vi "SVT Pumps Fans.vi"(0 "nominal speed [RPM]":dbl=1200.0, 1 "desired units":u16(ring) items=["Hz", "Order"], 5 "number of blades":u32=3, 7 "number of diffuser vanes":u32=10, 9 "blade length":dbl=1.0, 11 "error in (no error)":errorcluster) -> (3 "blade tip speed":dbl=62.83185307179586, 4 "blade pass frequency":dbl=60.0, 6 "blade rate frequency":dbl=600.0, 14 "common factor":i32=1, 15 "error out":errorcluster)   [LabVIEW 2017, in "SoundVib_MachineCharacteristic.lvlib"]
doc: "Calculates characteristic frequencies or orders of flow-induced machinery, such as pumps and fans."
uses:
  <vilib>/addons/Sound and Vibration/svt_Machine Characteristic/SoundVib_MachineCharacteristic.lvlib
  <vilib>/gmath/NI_Gmath.lvlib
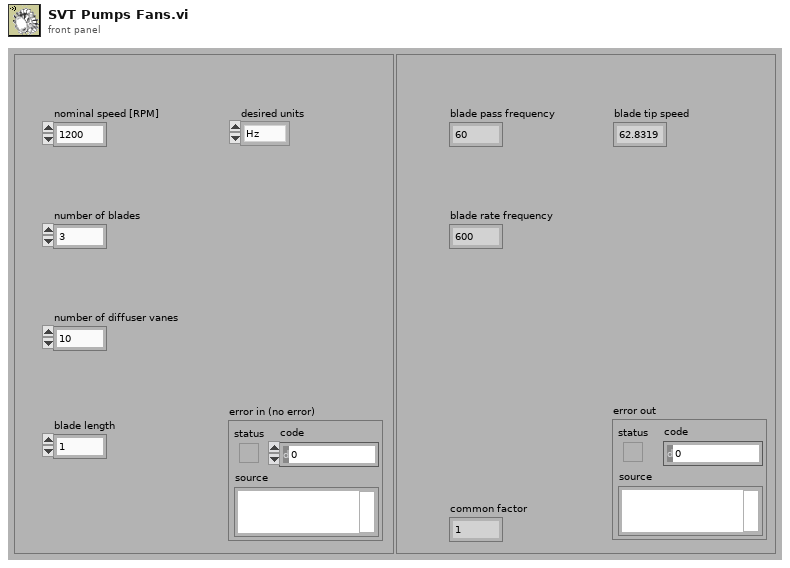
[diagram p1: front panel]
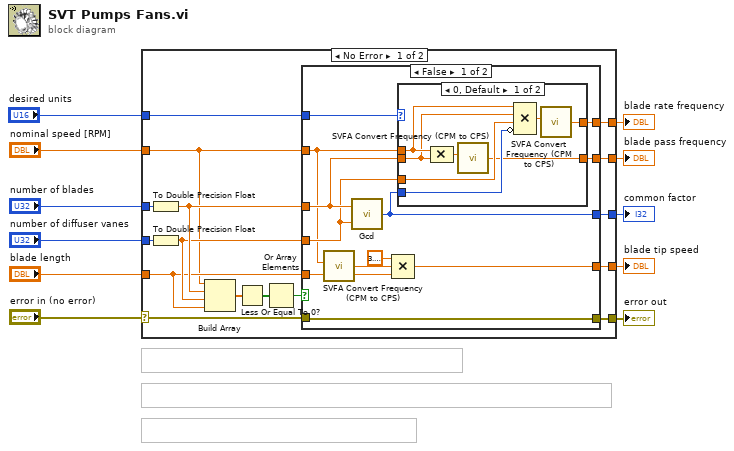
[diagram p0: block diagram]
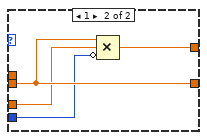
[diagram p2: hidden frame]
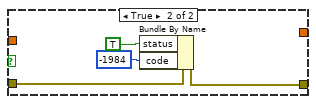
[diagram p3: hidden frame]
diagram:
  n1 = case shown="No Error" "error in (no error)" {
    selector: "error in (no error)" -> [w22 w56]
    tunnel: "blade length" -> [w18 _]
    tunnel: "number of diffuser vanes" -> [w27 _]
    tunnel: "number of blades" -> [w26 _]
    tunnel: "nominal speed [RPM]" -> [w15 _]
    tunnel: [w21 w56] -> w6
    tunnel: [w17 _] -> w5
    tunnel: "desired units" -> [w16 _]
    tunnel: [w14 _] -> w3
    tunnel: [w13 _] -> w2
    tunnel: [w12 _] -> w1
    frame No Error {
      n2 = To Double Precision Float(number=w26) -> (double precision float=w20:dbl)
      n3 = To Double Precision Float(number=w27) -> (double precision float=w19:dbl)
      n4 = Build Array(w15, w20, w19, w18) -> (w25:dbl[])
      n5 = Less Or Equal To 0?(x=w25) -> (x <= 0?=w24:bool[])
      n6 = Or Array Elements(Boolean array=w24) -> (logical OR=w23:bool)
      n7 = case shown="False" w23 {
        tunnel: w22 -> [w31 w55]
        tunnel: [w31 w54] -> w21
        tunnel: w20 -> [w38 _]
        tunnel: w19 -> [w37 _]
        tunnel: w18 -> [w33 _]
        tunnel: [w36 _] -> w17
        tunnel: w16 -> [w39 _]
        tunnel: w15 -> [w30 _]
        tunnel: [w35 _] -> w14
        tunnel: [w34 _] -> w13
        tunnel: [w28 _] -> w12
        frame False {
          n8 = call <vilib>:"SVFA Convert Frequency (CPM to CPS).vi"("nominal speed [RPM]"=w30) -> ("frequency [Hz]"=w29:dbl)  [unwired: 5 in]
          n9 = call <vilib>:"Gcd.vi"("y"=w37, "x"=w38) -> ("gcd(x,y)"=w36:i32)
          n10 = Compound Arithmetic op=MULTIPLY(3.141592653589793, w29, w33) -> (w28:dbl)
          n11 = case shown="0, Default" w39 {
            tunnel: w30 -> [w47 _]
            tunnel: w38 -> [w46 w51]
            tunnel: w37 -> [w45 w50]
            tunnel: w36 -> [w44 w48]
            tunnel: [w42 w51] -> w35
            tunnel: [w40 w49] -> w34
            frame 0, Default {
              n12 = Compound Arithmetic op=MULTIPLY(w47, w46) -> (w43:dbl)
              n13 = call <vilib>:"SVFA Convert Frequency (CPM to CPS).vi"("nominal speed [RPM]"=w43) -> ("frequency [Hz]"=w42:dbl)  [unwired: 5 in]
              n14 = Compound Arithmetic op=MULTIPLY(w47, w46, w45, invert w44) -> (w41:dbl)
              n15 = call <vilib>:"SVFA Convert Frequency (CPM to CPS).vi"("nominal speed [RPM]"=w41) -> ("frequency [Hz]"=w40:dbl)  [unwired: 5 in]
            }
            frame 1 {
              n16 = Compound Arithmetic op=MULTIPLY(w51, w50, invert w48) -> (w49:dbl)
            }
          }
        }
        frame True {
          n17 = Bundle By Name(cluster=w55, "status"=TRUE, "code"=-1984) -> (w54:errorcluster)
        }
      }
    }
    frame Error {
    }
  }
  "blade pass frequency" <- w3
  "error out" <- w6
  "blade rate frequency" <- w2
  "common factor" <- w5
  "blade tip speed" <- w1
